vi "IBM4_FR_Meas.vi"() -> ()   [LabVIEW 2020]
doc: "Rough and ready approach to automating FR measurement based on FHP code\n\nR. Sheehan 17 - 5 - 2021"
uses:
  LabVIEW/Common_VIs/Check_Range_Vals.vi
panel:
  out "Vin / V":dbl
  out "Vout / V":dbl
  out "Resp Plt":cluster{"Array":dbl[], "Array":dbl[]}(graph)
  out "Response":dbl
  out "fnow / kHz":dbl
  out "error out":errorcluster
  in  "error in (no error)":errorcluster
  in  "Addr In":refnum<visa-resource-name>="COM12"
  in  "df / kHz":dbl
  in  "fhi / kHz":dbl
  in  "flo / kHz":dbl
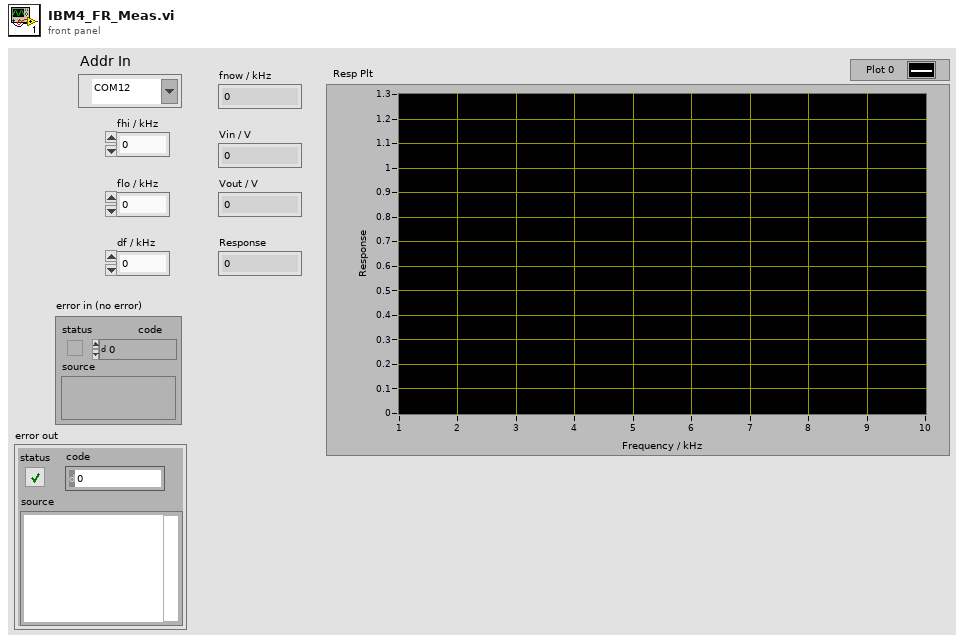
[diagram p1: front panel]
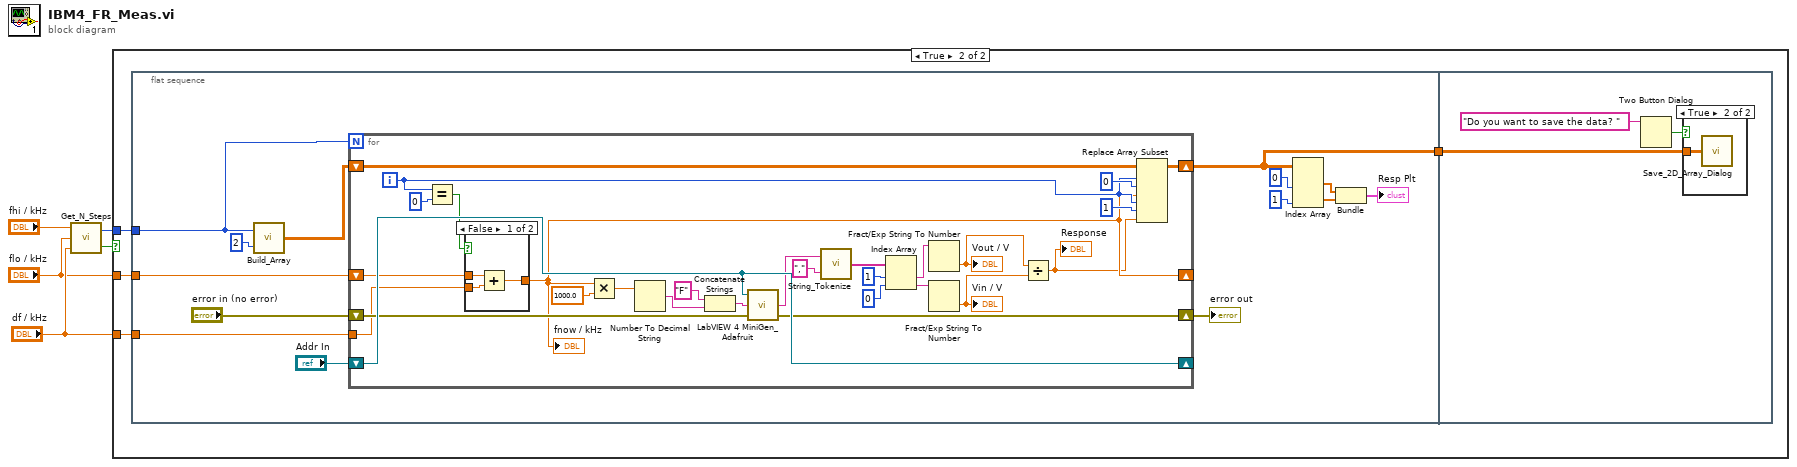
[diagram p0: block diagram]
diagram:
  n1 = call "Get_N_Steps.vi"("Increment"="df / kHz", "Lower Limit"="flo / kHz", "Upper Limit"="fhi / kHz") -> ("Bounds Are Good"=w4:bool, "N steps"=w1:i32)
  n2 = case shown="True" w4 {
    tunnel: "df / kHz" -> [_ w7]
    tunnel: "flo / kHz" -> [_ w8]
    tunnel: w1 -> [_ w9]
    frame False {
    }
    frame True {
      n3 = flat-sequence {
        tunnel: w9 -> [w23]
        tunnel: w8 -> [w17]
        tunnel: w7 -> [w16]
        tunnel: [w11] -> w6
        tunnel: w6 -> [w56]
        frame #0 {
          n4 = call "Build_Array.vi"("Ncolumns"=2, "Nrows"=w23) -> ("Array"=w21:dbl[][])
          n5 = for {
            N: w23 -> [_]
            shift-right: [w50] -> w11
            shift-left: w21 -> [w51]
            shift-right: [w47] -> _
            shift-left: "Addr In" -> [w47]
            shift-right: [w45] -> w18
            shift-left: "error in (no error)" -> [w46]
            tunnel: w16 -> [w40]
            shift-right: [w27] -> _
            shift-left: w17 -> [w41]
            i -> [w44]
            n6 = Equal?(x=w44, y=0) -> (x = y?=w42:bool)
            n7 = case shown="False" w42 {
              tunnel: w41 -> [w53 w55]
              tunnel: w40 -> [w54 _]
              tunnel: [w52 w55] -> w27
              frame False {
                n8 = Add(x=w53, y=w54) -> (x+y=w52:dbl)
              }
              frame True {
              }
            }
            "fnow / kHz" <- w27
            n9 = Multiply(x=w27, y=1000.0) -> (x*y=w37:dbl)
            n10 = Number To Decimal String(number=w37) -> (decimal integer string=w36:string)  [unwired: 1 in]
            n11 = Concatenate Strings("F" ("string"), w36) -> (w35:string)
            n12 = call "LabVIEW 4 MiniGen_Adafruit.vi"("error in (no error)"=w46, "write buffer"=w35, "VISA resource name"=w47) -> ("error out"=w45:errorcluster, "read buffer"=w33:string)  [unwired: 1 out]
            n13 = call "String_Tokenize.vi"("String Token"=",", "String"=w33) -> ("String Array"=w32:string[])
            n14 = Index Array(array=w32, index #1=1 ("index"), index #2=0 ("index")) -> (element #1=w29:string, element #2=w28:string)
            n15 = Fract/Exp String To Number(string=w29) -> (number=w25:dbl)  [unwired: 3 in, 1 out]
            "Vout / V" <- w25
            n16 = Fract/Exp String To Number(string=w28) -> (number=w24:dbl)  [unwired: 3 in, 1 out]
            "Vin / V" <- w24
            n17 = Divide(x=w25, y=w24) -> (x/y=w26:dbl)
            "Response" <- w26
            n18 = Replace Array Subset(array=w51, new element #1=w27, index (row) #1=w44, index (col) #1=0 ("disabled index (col)"), new element #2=w26, index (row) #2=w44, index (col) #2=1 ("index (col)")) -> (w50:dbl[][])
          }
          "error out" <- w18
          n19 = Index Array(array=w11, index (col) #1=0 ("disabled index (col)"), index (col) #2=1 ("index (col)")) -> (element #1=w13:dbl[], element #2=w12:dbl[])  [unwired: 2 in]
          n20 = Bundle("Array"=w13, "Array"=w12) -> (→"Resp Plt":cluster{"Array":dbl[], "Array":dbl[]})  [unwired: 1 in]
        }
        frame #1 {
          n21 = Two Button Dialog(message="Do you want to save the data? ") -> (T button?=w57:bool)  [unwired: 2 in]
          n22 = case shown="True" w57 {
            tunnel: w56 -> [_ w59]
            frame False {
            }
            frame True {
              n23 = call "Save_2D_Array_Dialog.vi"("2D data"=w59) -> ()
            }
          }
        }
      }
    }
  }
